vi "test.vi"() -> ()   [LabVIEW 2014]
uses:
  <vilib>/Utility/miscctls.llb/LVRectTypeDef.ctl
  <vilib>/Utility/miscctls.llb/LVPointTypeDef.ctl
  FT_HMI.llb/GLOBAL_GEN.vi
  ADS.llb/Global DIOs.vi
panel:
  in  "IMPRESSION OK":bool
  out "ST8_PRET_A_IMPRIMER":bool
  in  "stop":bool
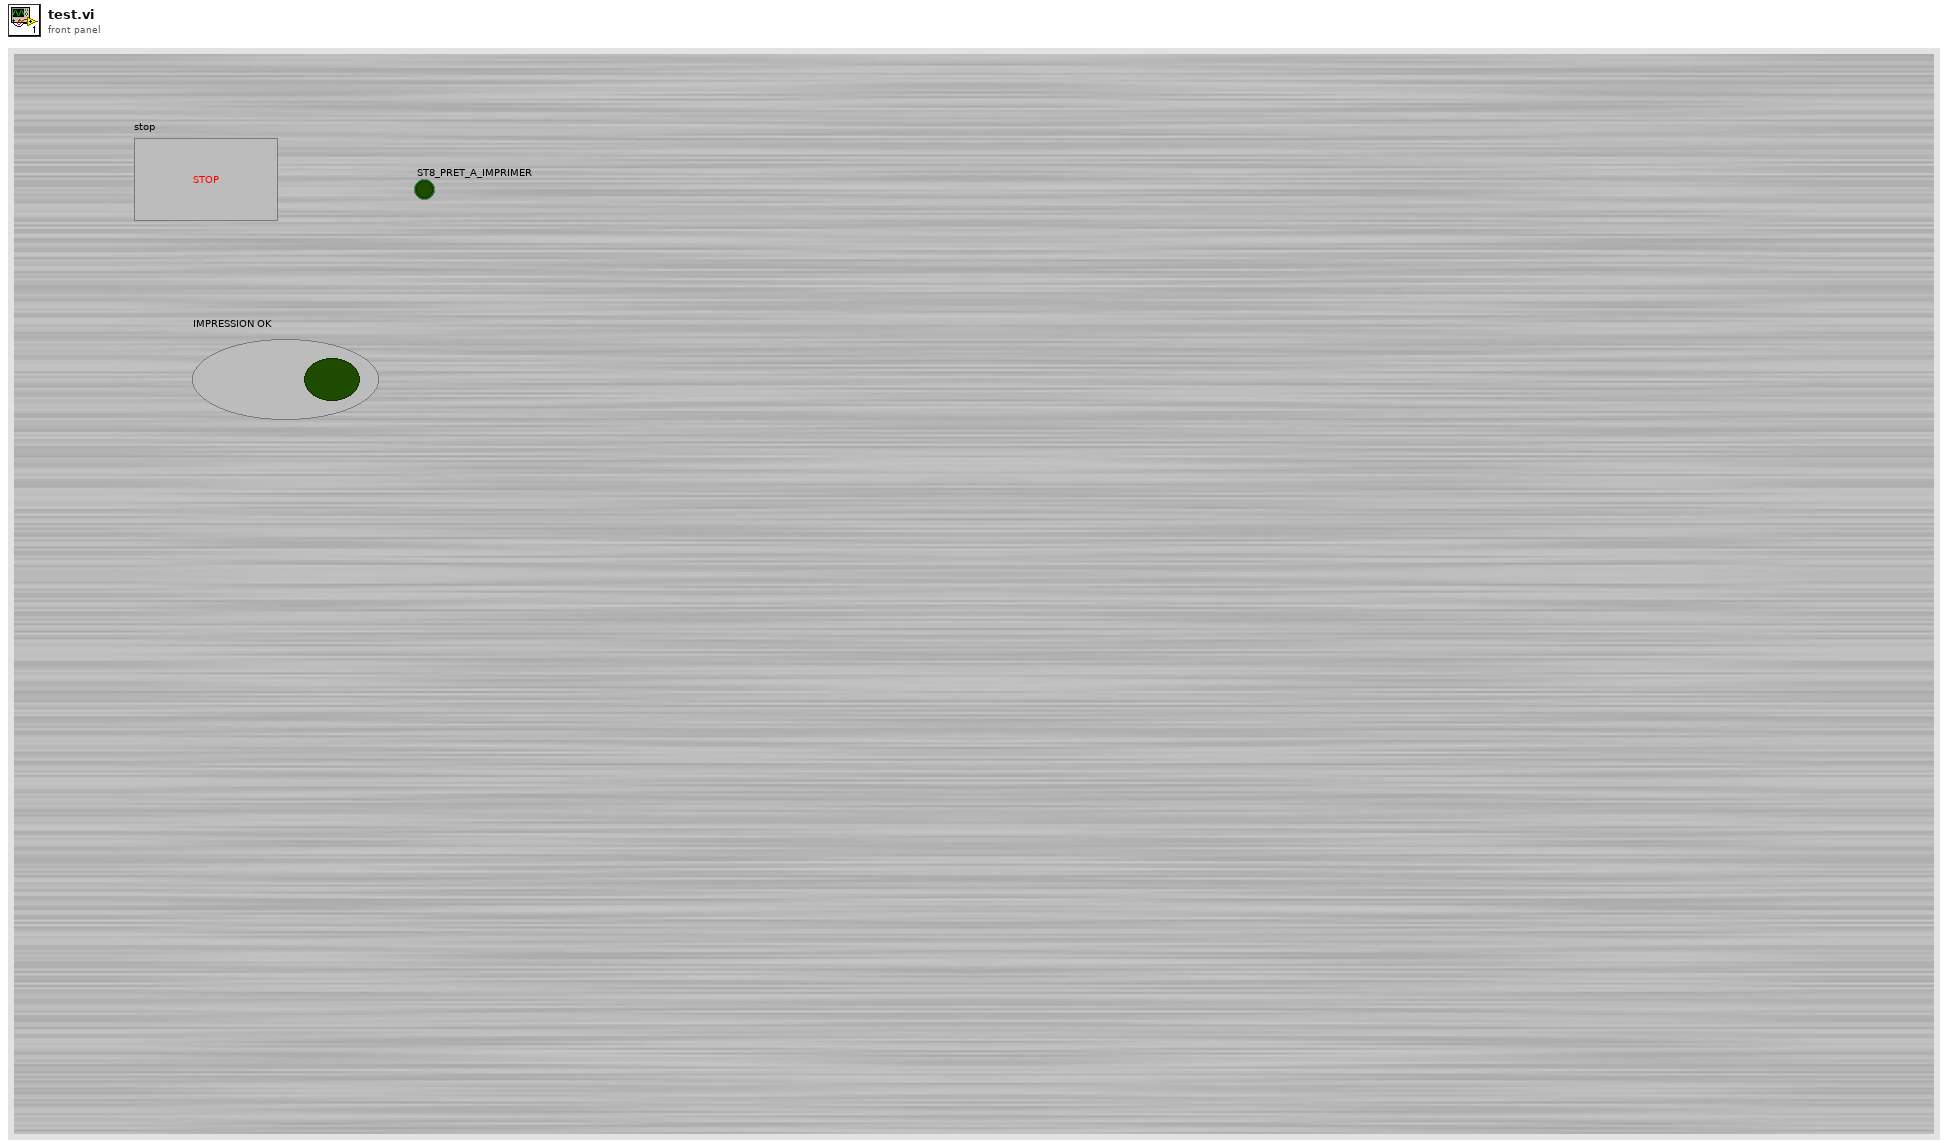
[diagram p1: front panel]
types:
  T1 = typedef "LVRectTypeDef.ctl" = cluster{"Left":i16, "Top":i16, "Right":i16, "Bottom":i16}
  T2 = typedef "LVPointTypeDef.ctl" = cluster{"Horizontal":i16, "Vertical":i16}
  T3 = cluster{"ADS_GEN_GRAND_DEBIT_Header":i32, "ADS_ST1_HT_NO_PROG_Header":i32, "ADS_ST2_TEMPS_POMPAGE_Header":i32, "ADS_ST2_CONTRE_PRESSION_Header":i32, "ADS_ST2_TEMPS_MESURE_Header":i32, "ADS_ST2_TEMPS_MESURE_PERTE_PRESSION_Header":i32, "ADS_ST3_TEMPS_MISE_SOUS_PRESSION_Header":i32, "ADS_ST3_TEMPS_STABILISATION_Header":i32, "ADS_ST3_TEMPS_MESURE_Header":i32, "ADS_ST45_TEMPS_POMPAGE_Header":i32, "ADS_ST45_TEMPS_MESURE_DEBIT_MAX_Header":i32, "ADS_ST45_PRESSION_CONSIGNE_Header":i32, "ADS_ST45_TEMPS_REGLAGE_PRESSION_Header":i32, "ADS_ST45_TEMPS_MESURE_DEBIT_Header":i32, "ADS_ST6_TEMPS_POMPAGE_Header":i32, "ADS_ST6_TEMPS_MESURE_Header":i32, "ADS_ST6_TEMPS_MESURE_PERTE_PRESSION_Header":i32, "ADS_SAFETY_EM_State_Header":i32, "ADS_FLAGS_INIT_Header":i32, "ADS_FLAGS_AUTO_Header":i32, "ADS_FLAGS_SAFETY_Header":i32, "ADS_RESET_EMERGENCY_Header":i32, "ADS_PROG_STEPS_Header":i32, "ADS_ST1_HT_OK_Header":i32, "ADS_ST8_PRET_A_IMPRIMER_Header":i32, "ADS_ST8_IMPRESSION_OK_Header":i32, "ADS_ST2_VACUUM_Header":i32, "ADS_ST3_DELTA_P_Header":i32, "ADS_ST45_QMAX_Header":i32, "ADS_ST45_Q_Header":i32, "ADS_ST45_PRESSURE_Header":i32, "ADS_ST45_COURANT_Header":i32, "ADS_ST45_VACUUM_Header":i32, "ADS_ST5_MODE_VIDANGE_Header":i16, "ADS_ST45_POIDS_Header":i32, "ADS_GEMMA_Header":i32, "ADS_ST7_TEMPS_SECHAGE_Header":i32, "ADS_ST9_BOBINE_A_FIL_Header":i32}
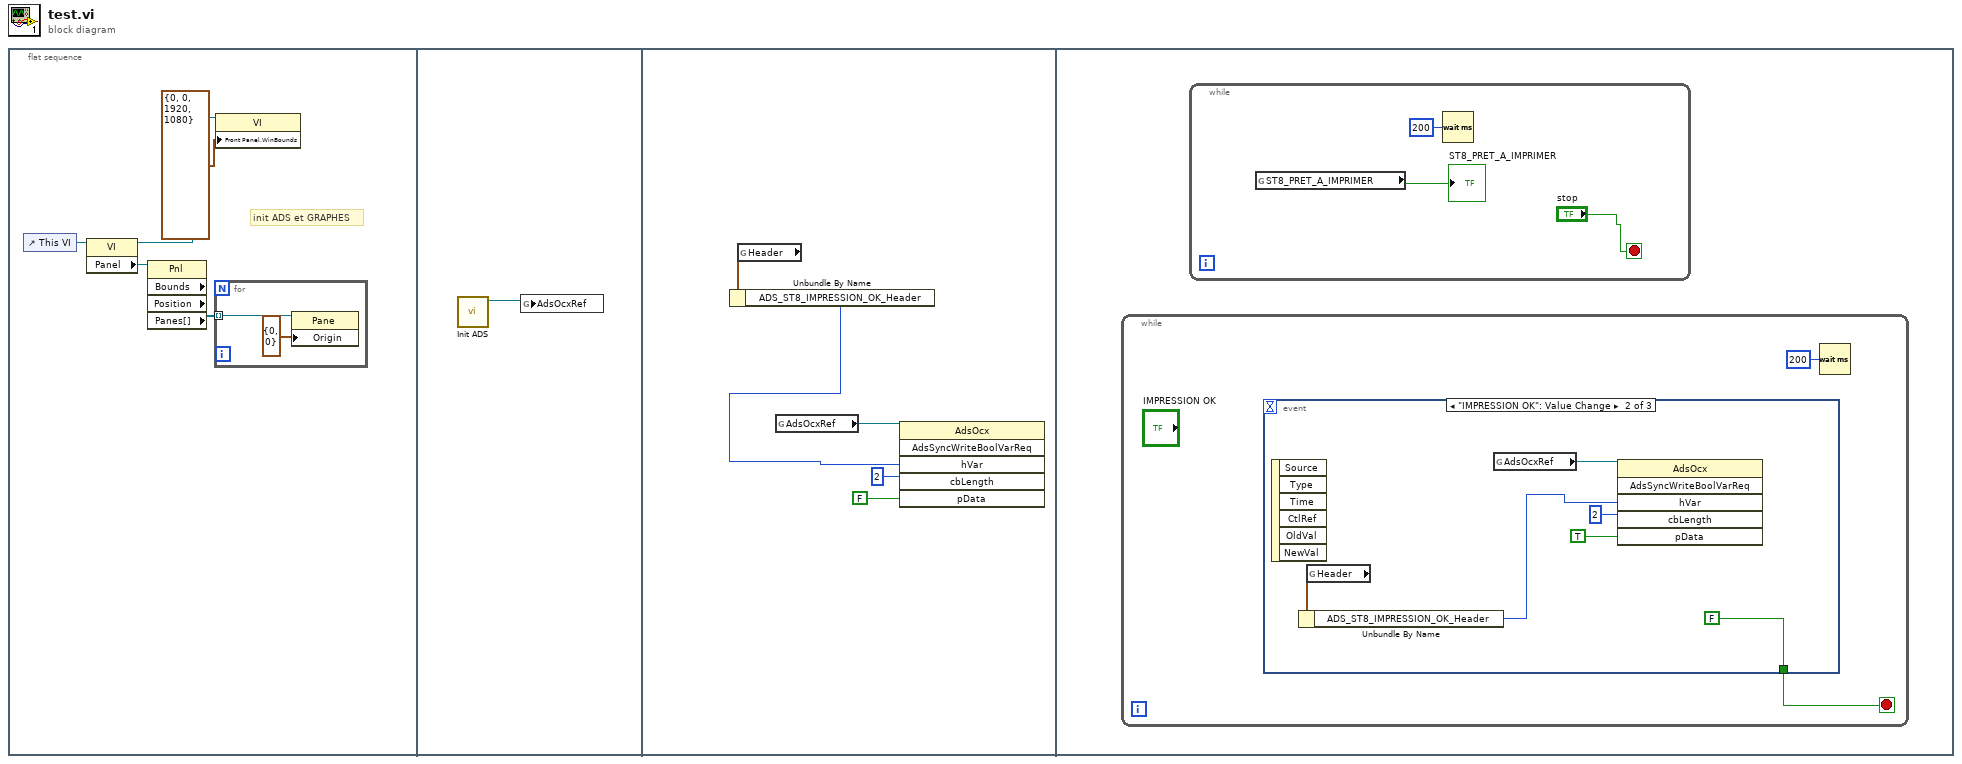
[diagram p0: block diagram]
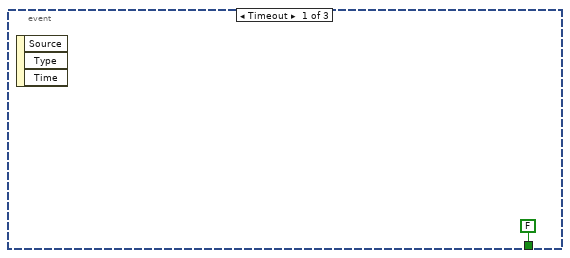
[diagram p2: hidden frame]
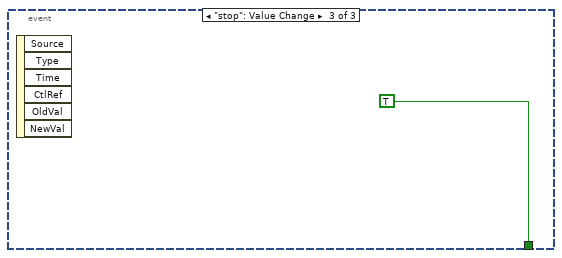
[diagram p3: hidden frame]
diagram:
  n1 = flat-sequence {
    frame #0 {
      # "init ADS et GRAPHES"
      n2 = control-ref of="This VI"() -> (w5:refnum<vi>)
      n3 = property class="VI"(reference=w5) -> (reference out=w4:refnum<vi>, "Panel"=w2:refnum<vi>)  [unwired: 1 in, 1 out]
      n4 = property class="Pnl" props=["Bounds", "Position", "Panes[]"](reference=w2) -> ("Panes[]"=w1:refnum<vi>[])  [unwired: 1 in, 4 out]
      n5 = for {
        tunnel: w1 -> [w6] mode=indexing
        n6 = property class="Pane"(reference=w6, "Origin"=T2 {"Horizontal"=0, "Vertical"=0}) -> ()  [unwired: 1 in, 2 out]
      }
      n7 = property class="VI"(reference=w4, "Front Panel.WinBounds"=T1 {"Left"=0, "Top"=0, "Right"=1920, "Bottom"=1080} ("Front Panel Window:Window Bounds")) -> ()  [unwired: 1 in, 2 out]
    }
    frame #1 {
      n8 = call "Init ADS.vi"() -> ("AdsOcxRef"=w8:refnum<k7>)  [unwired: 8 in, 1 out]
      n9 = global write "GLOBAL_GEN.vi" "AdsOcxRef"(w8) -> ()
    }
    frame #2 {
      n10 = global read "Global DIOs.vi" "Header"() -> (w10:T3)
      n11 = Unbundle By Name(w10) -> ("ADS_ST8_IMPRESSION_OK_Header"=w9:i32)
      n12 = global read "GLOBAL_GEN.vi" "AdsOcxRef"() -> (w13:refnum<k7>)
      n13 = invoke class="AdsOcx" method="AdsSyncWriteBoolVarReq"(reference=w13, "hVar"=w9, "cbLength"=2 ("phConnect"), "pData"=FALSE) -> ()  [unwired: 2 in, 6 out]
    }
    frame #3 {
      n14 = while {
        stop <- w15 stop-if-true
        n15 = event shown="[1] \"IMPRESSION OK\": Value Change" {
          selector: _ -> [_ _ _]
          dyn-events: _ -> [_ _ _]
          timeout: _ -> [_ _ _]
          tunnel: [FALSE ("pData") FALSE ("pData") TRUE ("pData")] -> w15
          event Timeout {
            n16 = event-data() -> ()  [unwired: 1 in, 3 out]
          }
          event "IMPRESSION OK": Value Change {
            n17 = event-data() -> ()  [unwired: 1 in, 6 out]
            n18 = global read "Global DIOs.vi" "Header"() -> (w18:T3)
            n19 = Unbundle By Name(w18) -> ("ADS_ST8_IMPRESSION_OK_Header"=w17:i32)
            n20 = global read "GLOBAL_GEN.vi" "AdsOcxRef"() -> (w21:refnum<k7>)
            n21 = invoke class="AdsOcx" method="AdsSyncWriteBoolVarReq"(reference=w21, "hVar"=w17, "cbLength"=2 ("phConnect"), "pData"=TRUE) -> ()  [unwired: 2 in, 6 out]
          }
          event "stop": Value Change {
            n22 = event-data() -> ()  [unwired: 1 in, 6 out]
          }
        }
        n23 = Wait (ms)(milliseconds to wait=u32 200) -> ()  [unwired: 1 out]
      }
      n24 = while {
        stop <- "stop" stop-if-true
        n25 = global read "Global DIOs.vi" "ST8_PRET_A_IMPRIMER"() -> (→"ST8_PRET_A_IMPRIMER":bool)
        n26 = Wait (ms)(milliseconds to wait=u32 200) -> ()  [unwired: 1 out]
      }
    }
  }
